vi "SSL Detection Frame Robots Kalman Estimator VelCmd.vi"(0 "Lado":enum16{"Esquerdo", "Direito"}(ring) caption="Enum", 5 "Time Stamp":timestamp, 6 "our_robots":bool=TRUE, 7 "Life Time":dbl=1.0, 8 "ignora esquerda?":bool=TRUE, 9 "ignora lado":bool, 10 "our_robots":T1[](array[typedef]), 11 "Robots":T6[](array[typedef]) {"height" format="%+4.3f"; "pixel_y" format="%+4.3f"; "pixel_x" format="%+4.3f"; "orientation" format="%+4.3f"; "y" format="%+4.3f"; "confidence" format="%4.3f"; "x" format="%+4.3f"}) -> (3 "Robots Out":T6[](array[typedef]) {"height" format="%+4.3f"; "pixel_y" format="%+4.3f"; "pixel_x" format="%+4.3f"; "orientation" format="%+4.3f"; "y" format="%+4.3f"; "confidence" format="%4.3f"; "x" format="%+4.3f"})   [LabVIEW 2017]
uses:
  SSL Detection Robot.ctl
  <vilib>/Analysis/Matrix/Datatypes/RealMatrix.ctl
  Core/AI Robot.ctl
  Intel/Functions Enum.ctl
  Intel/AttackerStates.ctl
  Path Planning/RRT/PathDests.ctl
  Path Planning/RRT/PathDest.ctl
  <vilib>/Analysis/coordinate.llb/Wrap Angle (scalar).vi
  <vilib>/Analysis/_algsub.llb/Real Vector Norm.vi
  <vilib>/Analysis/Matrix/Numeric/Conversions/Array To Matrix - RA.vi
  <vilib>/Analysis/Matrix/Numeric/Subtract/Subtract - RM,RM.vi
  <vilib>/Analysis/NI_AALPro.lvlib
  <vilib>/Analysis/Matrix/NI_Matrix.lvlib
  <vilib>/Analysis/NI_AAL_Angle.lvlib
panel:
  in  "Robots Out 2":T8(array[cluster]) {"Detection Robot"."height" format="%+4.3f"; "Detection Robot"."pixel_y" format="%+4.3f"; "Detection Robot"."pixel_x" format="%+4.3f"; "Detection Robot"."orientation" format="%+4.3f"; "Detection Robot"."y" format="%+4.3f"; "Detection Robot"."confidence" format="%4.3f"; "Detection Robot"."x" format="%+4.3f"}
  out "A-B":dbl[][](array[numeric])
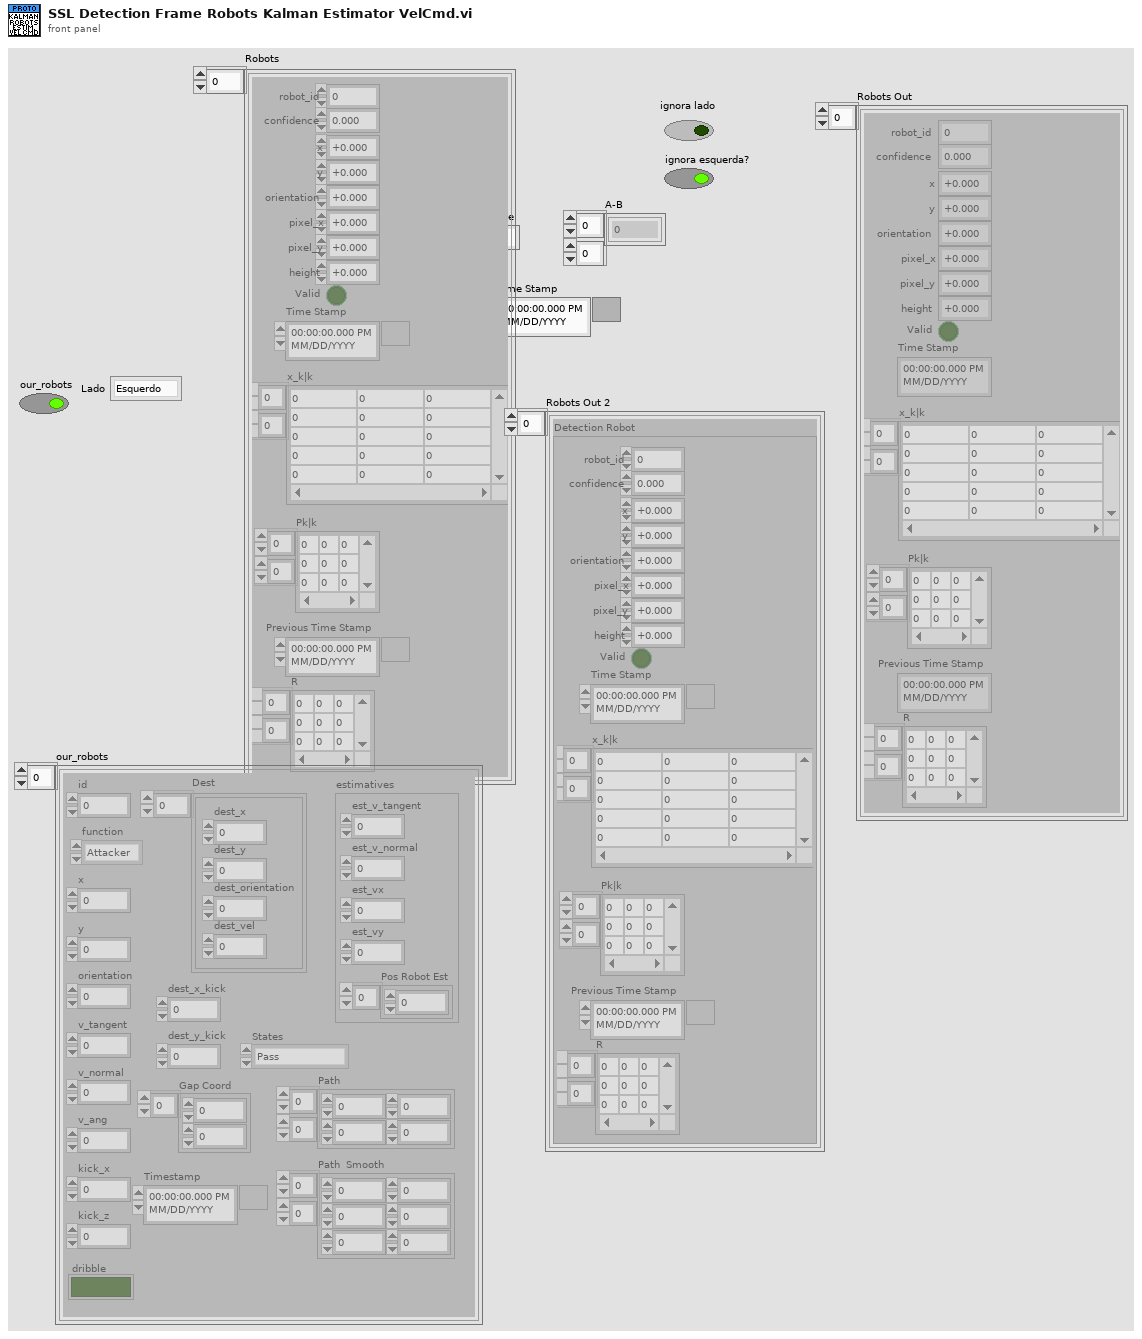
[diagram p1: front panel]
types:
  T1 = typedef "AI Robot.ctl" = cluster{"id":u32, "function":T2, "x":dbl, "y":dbl, "orientation":dbl, "v_tangent":dbl, "v_normal":dbl, "v_ang":dbl, "kick_x":dbl, "kick_z":dbl, "dribble":bool, "Timestamp":timestamp, "estimatives":cluster{"est_v_tangent":dbl, "est_v_normal":dbl, "est_vx":dbl, "est_vy":dbl, "Pos Robot Est":dbl[]}, "dest_x_kick":dbl, "dest_y_kick":dbl, "Gap Coord":dbl[], "States":T3, "Path ":dbl[][], "Path  Smooth":dbl[][], "Dest":T4}
  T2 = typedef "Functions Enum.ctl" = enum16{"Attacker", "Goalie", "Defender", "Striker", "Goto 0", "Dummy", "Kicker", "ZigZag"}
  T3 = typedef "AttackerStates.ctl" = enum16{"Pass", "GoToTangent", "BallGetting", "GoToKick", ""}
  T4 = typedef "PathDests.ctl" = T5[]
  T5 = typedef "PathDest.ctl" = cluster{"dest_x":dbl, "dest_y":dbl, "dest_orientation":dbl, "dest_vel":dbl}
  T6 = typedef "SSL Detection Robot.ctl" = cluster{"x":sgl, "robot_id":u32, "confidence":sgl, "y":sgl, "orientation":sgl, "pixel_x":sgl, "pixel_y":sgl, "height":sgl, "Valid":bool, "Time Stamp":timestamp, "x_k|k":T7, "Pk|k":T7, "Previous Time Stamp":timestamp, "R":T7}
  T7 = typedef "NI_Matrix.lvlib/RealMatrix.ctl" = dbl[][]
  T8 = cluster{"Detection Robot":T6, "Real Matrix (Column Vector)":T7, "Pk|k":T7}[]
  T9 = cluster{"Detection Robot":T6, "Real Matrix (Column Vector)":T7, "Pk|k":T7}
  T10 = cluster{"Detection Robot out":T6, "x_k|k":T7, "Pk|k":T7}
  T11 = typedef "SSL Detection Robot.ctl" = cluster{"x":sgl, "robot_id":u32, "confidence":sgl, "y":sgl, "orientation":sgl, "pixel_x":sgl, "pixel_y":sgl, "height":sgl, "Valid":bool, "Time Stamp":timestamp, "x_k|k":T7, "Pk|k":T7}
  T12 = cluster{"Detection Robot":T11, "Real Matrix (Column Vector)":T7, dbl[][]}
  T13 = cluster{"Detection Robot out":T6, "x_k|k":T7, "Pk|k":T7}[]
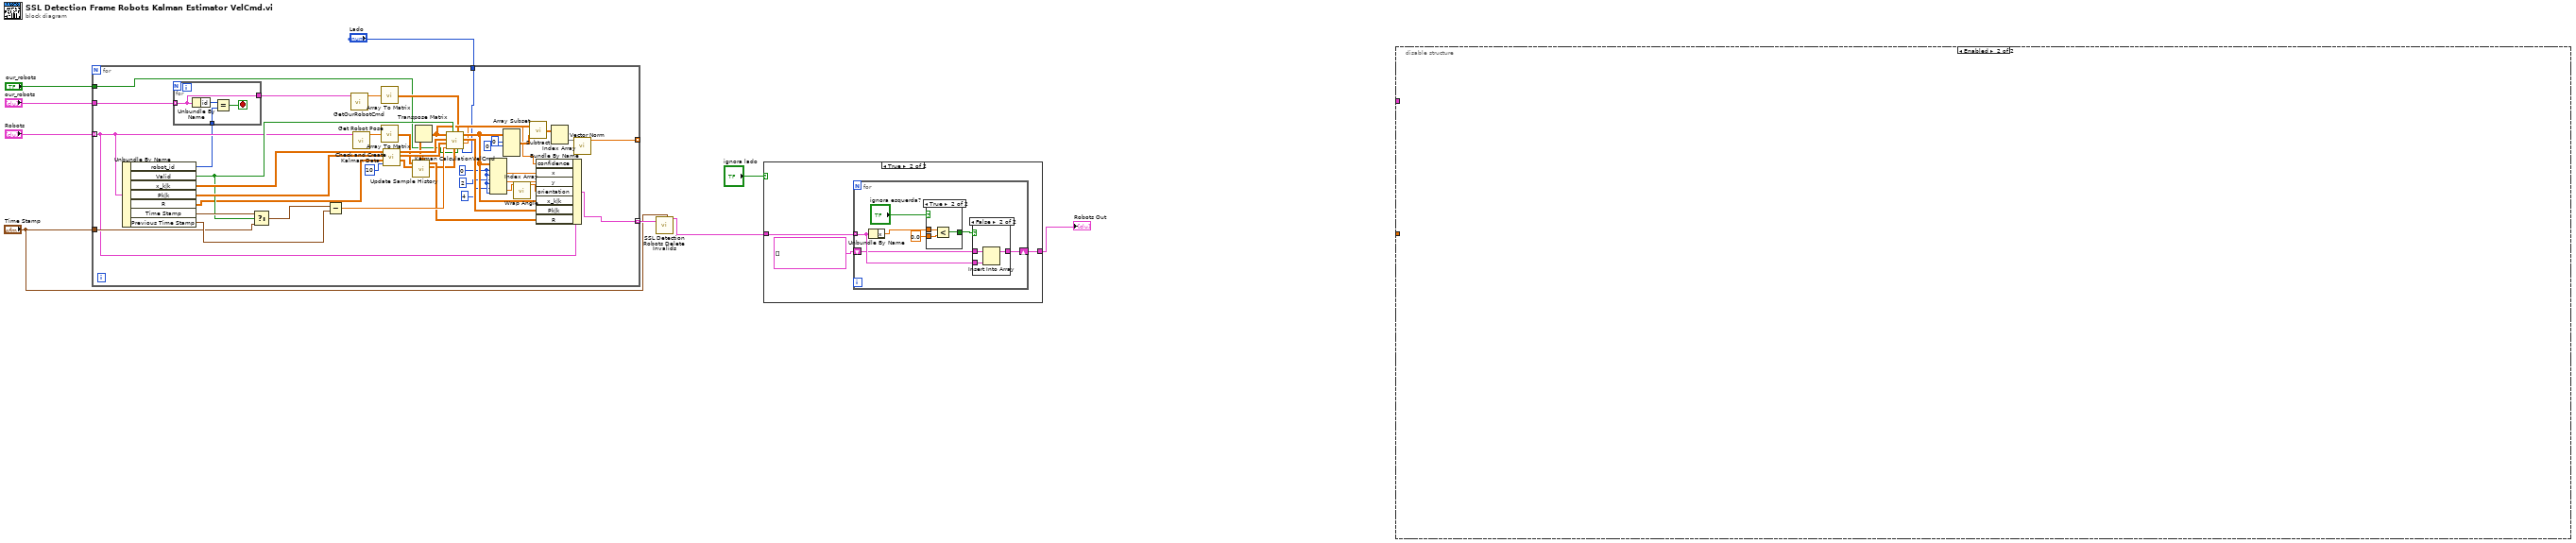
[diagram p0: block diagram]
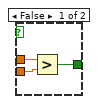
[diagram p3: hidden frame]
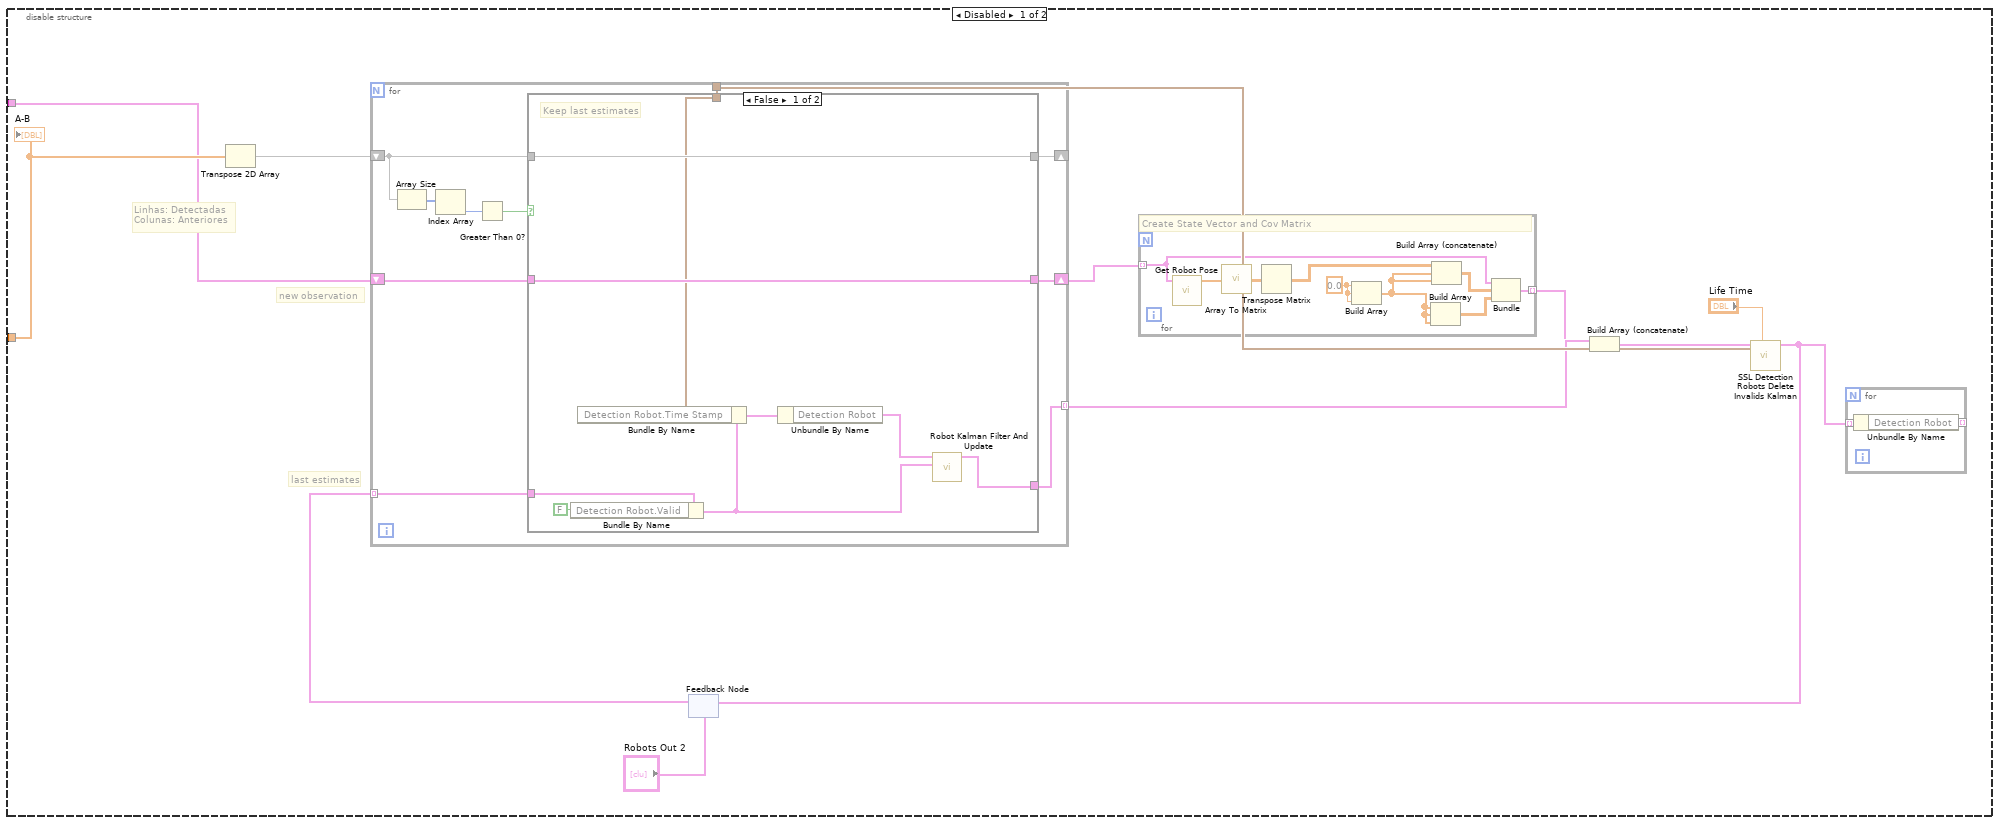
[diagram p5: hidden frame]
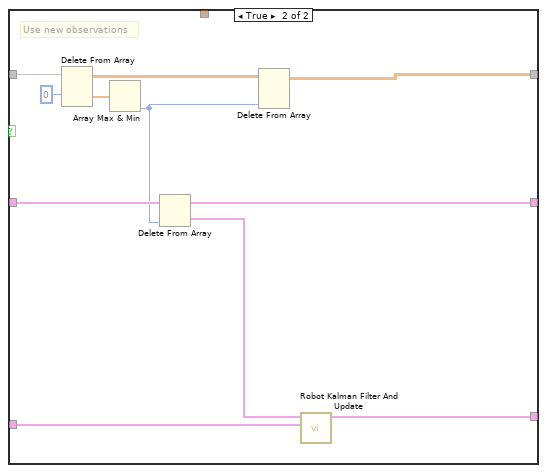
[diagram p6: hidden frame]
diagram:
  n1 = for {
    tunnel: "Robots" -> [w35] mode=indexing
    tunnel: [w53] -> _ mode=indexing
    tunnel: [w17] -> w8 mode=indexing
    tunnel: "Time Stamp" -> [w38]
    tunnel: "our_robots" -> [w16]
    tunnel: "our_robots" -> [w11]
    tunnel: "Lado" -> [w10]
    w31 = 0 ("index (row)")
    n2 = Unbundle By Name(w35) -> ("robot_id"=w15:u32, "Valid"=w36:bool, "x_k|k"=w45:T7, "Pk|k"=w43:T7, "R"=w28:T7, "Time Stamp"=w39:timestamp, "Previous Time Stamp"=w41:timestamp)
    n3 = for {
      tunnel: w16 -> [w54] mode=indexing
      tunnel: w15 -> [w55]
      tunnel: [w54] -> w14
      stop <- w57 stop-if-true
      n4 = Unbundle By Name(w54) -> ("id"=w56:u32)
      n5 = Equal?(x=w56, y=w55) -> (x = y?=w57:bool)
    }
    n6 = Select(t=w39, s=w36, f=w38) -> (s? t:f=w37:timestamp)
    n7 = Subtract(x=w37, y=w41) -> (x-y=w40:dbl)
    n8 = call "GetOurRobotCmd.vi"("Robot"=w14) -> ("Vel"=w13:dbl[])  [unwired: 10 in]
    n9 = call "Get Robot Pose.vi"("Detection Robot"=w35) -> ("Pose"=w47:sgl[])  [unwired: 10 in]
    n10 = call-poly <vilib>:"Array To Matrix.vi"("Real 1D Array"=w13) -> ("Real Matrix (Column Vector)"=w12:T7)
    n11 = call-poly <vilib>:"Array To Matrix.vi"("Real 1D Array"=w47) -> ("Real Matrix (Column Vector)"=w24:T7)
    n12 = call "Check and Create Kalman Data.vi"("Variance Memory"=10, "R"=w28, "Pk"=w43, "x_k"=w45) -> ("R out"=w27:T7, "Pk out"=w42:T7, "x_k out"=w44:T7)  [unwired: 5 in]
    n13 = call "Update Sample History.vi"("R in"=w27, "Sample"=w24) -> ("covariance matrix V"=w22:T7, "R out"=w23:T7, "Sample Unwrapped"=w21:T7)  [unwired: 7 in]
    n14 = Transpose Matrix(1:w21) -> (0:w25:T7)
    n15 = call "Kalman CalculationVelCmd.vi"("Lado"=w10, "our_robots"=w11, "u_k"=w12, "R"=w22, "Use Observation"=w36, "intervalo"=w40, "Pk-1|k-1"=w42, "x_k-1|k-1"=w44, "z_k"=w25) -> ("Conf"=w18:dbl, "Pk|k"=w46:T7, "x_k|k"=w34:T7)
    n16 = Index Array(array=w34, index (row) #1=w31, index (col) #1=w31, index (row) #2=2 ("disabled index (col)"), index (col) #2=w31, index (row) #3=4 ("disabled index (col)"), index (col) #3=w31) -> (element #1=w33:dbl, element #2=w32:dbl, element #3=w20:dbl)
    n17 = Array Subset(array=w34, index (row)=0 ("row 1"), length (row)=0 ("row N")) -> (w52:T7)  [unwired: 2 in]
    n18 = call-poly <vilib>:"Wrap Angle.vi"("angle in"=w20) -> ("angle out"=w19:dbl)  [unwired: 9 in, 1 out]
    n19 = call-poly <vilib>:"Subtract.vi"("Real Matrix B"=w52, "Real Matrix A"=w25) -> ("A - B"=w49:T7)
    n20 = Bundle By Name(cluster=w35, "confidence"=w18, "x"=w33, "y"=w32, "orientation"=w19, "x_k|k"=w34, "Pk|k"=w46, "R"=w23) -> (w17:T6)
    n21 = Index Array(array=w49) -> (element=w48:dbl[])  [unwired: 2 in]
    n22 = call-poly <vilib>:"Vector Norm.vi"("Input Vector"=w48) -> ("norm"=w53:dbl)  [unwired: 9 in, 1 out]
  }
  n23 = call "SSL Detection Robots Delete Invalids.vi"("Now"="Time Stamp", "Robots In"=w8) -> ("Robots Out"=w5:T6[])  [unwired: 9 in]
  n24 = case shown="True" "ignora lado" {
    tunnel: w5 -> [w58 w61]
    tunnel: [w58 w59] -> w4
    frame False {
    }
    frame True {
      n25 = for {
        tunnel: w61 -> [w68] mode=indexing
        shift-right: [w62] -> w59
        shift-left: T6[] [] ("Robots Out") -> [w63]
        n26 = Unbundle By Name(w68) -> ("x"=w67:sgl)
        n27 = case shown="True" "ignora esquerda?" {
          tunnel: w67 -> [w71 w74]
          tunnel: sgl 0.0 ("y") -> [w70 w73]
          tunnel: [w69 w72] -> w65
          frame False {
            n28 = Greater?(x=w71, y=w70) -> (0:w69:bool)
          }
          frame True {
            n29 = Less?(x=w74, y=w73) -> (x < y?=w72:bool)
          }
        }
        n30 = case shown="False" w65 {
          tunnel: w68 -> [_ w77]
          tunnel: [w75 w78] -> w62
          tunnel: w63 -> [w75 w76]
          frame True {
          }
          frame False {
            n31 = Insert Into Array(array=w76, new element=w77) -> (w78:T6[])  [unwired: 1 in]
          }
        }
      }
    }
  }
  "Robots Out" <- w4
  n32 = disable-structure shown="Enabled" {
    disable-tunnel: _ -> [w87 _]
    disable-tunnel: _ -> [w86 _]
    frame Disabled {
      # "Linhas: Detectadas\nColunas: Anteriores"
      # "last estimates"
      # "new observation"
      n33 = Transpose 2D Array(2D array=w87) -> (transposed array=w88:dbl[][])
      n34 = feedback #1("Robots Out 2") -> (w80:T8)
      n35 = for {
        shift-right: [w110] -> _
        shift-left: w88 -> [w106]
        shift-right: [w109] -> w85
        shift-left: w86 -> [w111]
        tunnel: [w108] -> w84 mode=indexing
        tunnel: w80 -> [w107] mode=indexing
        tunnel: [w102] -> w89
        n36 = Array Size(array=w106) -> (size(s)=w104:i32[])
        n37 = Index Array(array=w104) -> (element=w103:i32)  [unwired: 1 in]
        n38 = Greater Than 0?(x=w103) -> (x > 0?=w105:bool)
        n39 = case shown="False" w105 {
          tunnel: w106 -> [w120 w131]
          tunnel: w111 -> [w119 w128]
          tunnel: [w120 w126] -> w110
          tunnel: [w119 w124] -> w109
          tunnel: [w115 w123] -> w108
          tunnel: w107 -> [w114 w121]
          tunnel: w102 -> [w117 _]
          frame False {
            # "Keep last estimates"
            n40 = Bundle By Name(cluster=w114, "Detection Robot.Valid"=FALSE ("Detection Ball.Valid")) -> (w112:T9)
            n41 = Bundle By Name(cluster=w112, "Detection Robot.Time Stamp"=w117) -> (w116:T9)
            n42 = Unbundle By Name(w116) -> ("Detection Robot"=w113:T6)
            n43 = call "Robot Kalman Filter And Update.vi"("Cluster in"=w112, "Detection Robot"=w113) -> ("Cluster out"=w115:T10)  [unwired: 9 in]
          }
          frame True {
            # "Use new observations"
            n44 = Delete From Array(array=w131, index (row)=0) -> (deleted portion=w129:dbl[], array with subset deleted=w127:dbl[][])  [unwired: 2 in]
            n45 = Array Max & Min(array=w129) -> (min index (indices)=w125:i32)  [unwired: 3 out]
            n46 = Delete From Array(array=w128, index=w125) -> (deleted portion=w122:T11, array with subset deleted=w124:T11[])  [unwired: 1 in]
            n47 = Delete From Array(array=w127, index (col)=w125) -> (array with subset deleted=w126:dbl[][])  [unwired: 2 in, 1 out]
            n48 = call "Robot Kalman Filter And Update.vi"("Cluster in"=w121, "Detection Robot"=w122) -> ("Cluster out"=w123:T10)  [unwired: 9 in]
          }
        }
      }
      n49 = for {
        tunnel: w85 -> [w94] mode=indexing
        tunnel: [w97] -> w83 mode=indexing
        w101 = 0.0 ("element")
        # "Create State Vector and Cov Matrix"
        n50 = call "Get Robot Pose.vi"("Detection Robot"=w94) -> ("Pose"=w96:sgl[])  [unwired: 10 in]
        n51 = call-poly <vilib>:"Array To Matrix.vi"("Real 1D Array"=w96) -> ("Real Matrix (Column Vector)"=w95:T7)
        n52 = Transpose Matrix(1:w95) -> (0:w93:T7)
        n53 = Build Array(w101, w101, w101) -> (w100:dbl[])
        n54 = Build Array(w100, w100, w100) -> (w99:dbl[][])
        n55 = Build Array (concatenate)(w93, w100, w100) -> (w98:T7)
        n56 = Bundle("Detection Robot"=w94, "Real Matrix (Column Vector)"=w98, w99) -> (w97:T12)  [unwired: 1 in]
      }
      n57 = Build Array (concatenate)(w84, w83) -> (w79:T13)
      n58 = call "SSL Detection Robots Delete Invalids Kalman.vi"("Now"=w89, "Life Time"="Life Time", "Robots In"=w79) -> ("Robots Out"=w82:T8)  [unwired: 8 in]
      n59 = feedback-in #1(w82) -> ()
      n60 = for {
        tunnel: w82 -> [w92] mode=indexing
        tunnel: [w91] -> _ mode=indexing
        n61 = Unbundle By Name(w92) -> ("Detection Robot"=w91:T6)
      }
      "A-B" <- w87
    }
    frame Enabled {
    }
  }
